vi "remove zero from array.vi"(10 "in":dbl[](array[numeric])) -> (2 "out":dbl[](array[numeric]))   [LabVIEW 2024]
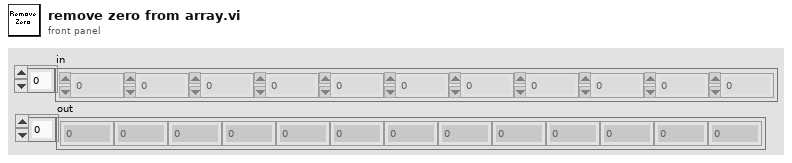
[diagram p1: front panel]
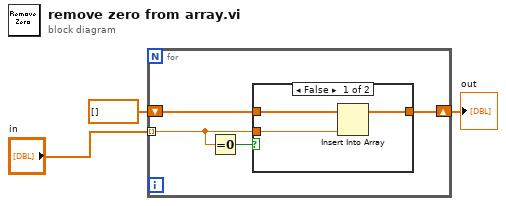
[diagram p0: block diagram]
diagram:
  n1 = for {
    tunnel: "in" -> [w7] mode=indexing
    shift-right: [w4] -> w1
    shift-left: dbl[] [] -> [w5]
    n2 = Equal To 0?(x=w7) -> (x = 0?=w6:bool)
    n3 = case shown="False" w6 {
      tunnel: [w8 w11] -> w4
      tunnel: w7 -> [w9 _]
      tunnel: w5 -> [w10 w11]
      frame False {
        n4 = Insert Into Array(array=w10, new element=w9) -> (w8:dbl[])  [unwired: 1 in]
      }
      frame True {
      }
    }
  }
  "out" <- w1
